vi "Add Point Procedural.vi"(4 "New X":i32, 6 "New Y":i32, 8 "Memory allocated in":i32, 9 "Number of points in":i32, 10 "Y Values in":i32[](array[numeric]), 11 "X Values in":i32[](array[numeric])) -> (0 "Memory allocated out":i32, 1 "Number of Points out":i32, 2 "Y Values out":i32[](array[numeric]), 3 "X Values out":i32[](array[numeric]))   [LabVIEW 2013, in "Outline.lvclass"]
doc: "Provides massive speedup over Add Point, object oriented for large numbers of runs. There appears to be a large overhead for object methods. Making an object oriented routine a subroutine does not fix this. This problem exists in labview 8.2."
uses:
  Outline.lvclass
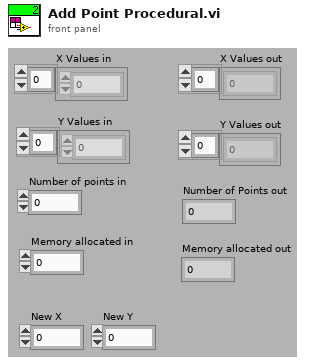
[diagram p1: front panel]
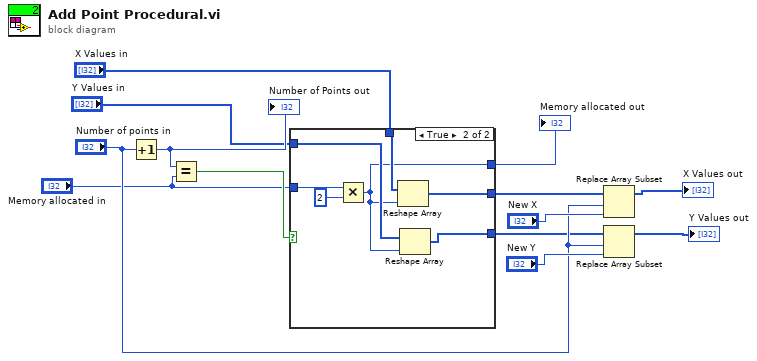
[diagram p0: block diagram]
diagram:
  n1 = Increment(x="Number of points in") -> (x+1=w10:i32)
  "Number of Points out" <- w10
  n2 = Equal?(x=w10, y="Memory allocated in") -> (x = y?=w3:bool)
  n3 = case shown="True" w3 {
    tunnel: "X Values in" -> [w16 w23]
    tunnel: "Memory allocated in" -> [w14 w22]
    tunnel: "Y Values in" -> [w15 w20]
    tunnel: [w16 w19] -> w5
    tunnel: [w15 w18] -> w6
    tunnel: [w14 w17] -> w11
    frame False {
    }
    frame True {
      n4 = Multiply(x=w22, y=2) -> (x*y=w17:i32)
      n5 = Reshape Array(w23, w17) -> (w19:i32[])
      n6 = Reshape Array(w20, w17) -> (w18:i32[])
    }
  }
  "Memory allocated out" <- w11
  n7 = Replace Array Subset(array=w5, new element="New X", index="Number of points in") -> (→"X Values out":i32[])
  n8 = Replace Array Subset(array=w6, new element="New Y", index="Number of points in") -> (→"Y Values out":i32[])
